vi "Programa Vent.vi"() -> ()   [LabVIEW 2021]
uses:
  4c7040a6-f012-4fa6-bc11-eaa48d4a9fce.vi
  <vilib>/Instr/_visa.llb/VISA Configure Serial Port (Instr).vi
panel:
  out "FLUJO":waveform(dbl)(graph)
  in  "Caract. Escalon":bool
  in  "Caract. Rampa":bool
  in  "Comenzar Caracterizacion":bool
  out "VIF":i16=211
  out "VEF":i16=1
  out "PIP":i16=1
  out "BPM":i16=7
  out "T Ciclo Resp.":dbl=9.2 format="%#_2g"
  in  "Modo Asistido":bool
  out "Fecha y Hora":timestamp=timestamp(3714054510.5922894 s since 1904-01-01) format="%<%X\n%x>T"
  out "PRESIÓN":waveform(dbl)(graph)
  in  "T. Espiración (s)":dbl=3.0 min=1.0 max=5.0 step=0.25
  in  "T. Plateau (s)":dbl=0.5 min=0.0 max=1.0 step=0.1
  in  "Comenzar Respiración":bool
  in  "Volumen deseado":dbl=350.0 min=100.0 max=2000.0 step=10.0
  in  "Presión Soporte\n (Volumen control)":dbl=20.0 min=10.0 max=60.0 step=1.0
  in  "PEEP deseado":dbl=5.0 min=0.0 max=20.0 step=1.0
  in  "Porcentaje Válvula":dbl=50.0 min=0.0 max=100.0 step=1.0
  out "Serial Write":string="0.000000,50.000000,20.000000,5.000000,350.000000,3000.000000,500.000000,0.000000,0.000000,0.000000,0.000000\r\n"
  out "Volumen-Ins":i16=211
  out "Flujo":i16
  out "PEEP":i16=4
  out "Serial Read":string="Presion: 1.42,Peep: 3.57,Presion_soporte: 20,Flujo: -0.35,Volumen deseado: 350, Volumen inspiracion: 211.01,PIP: 1.00,VEF: 1.00,VIF: 211.00,T_muestreo: 4.00, PWM Out: 5000, Timer_Count_0: 0, Etapa_Res: 0, Derivada_Presion: 0.00, duracion_ciclo: 9200.00, BPM: 6.52, PWM_Caract: 0, T. Trans_Caract: 0.00, MV: 0.00, String: 0.000000,50.000000,20.000000,5.000000,350.000000,3000.000000,500.000000,0.000000,0.000000,0.000000,0.000000\r\r\n"
  in  "stop":bool
  # "Ventilador Mecánico de Emergencia"
  # "Modo de Operación"
  # "Volumen\nControl"
  # "GRÁFICOS"
  # "Seccion de Datos:"
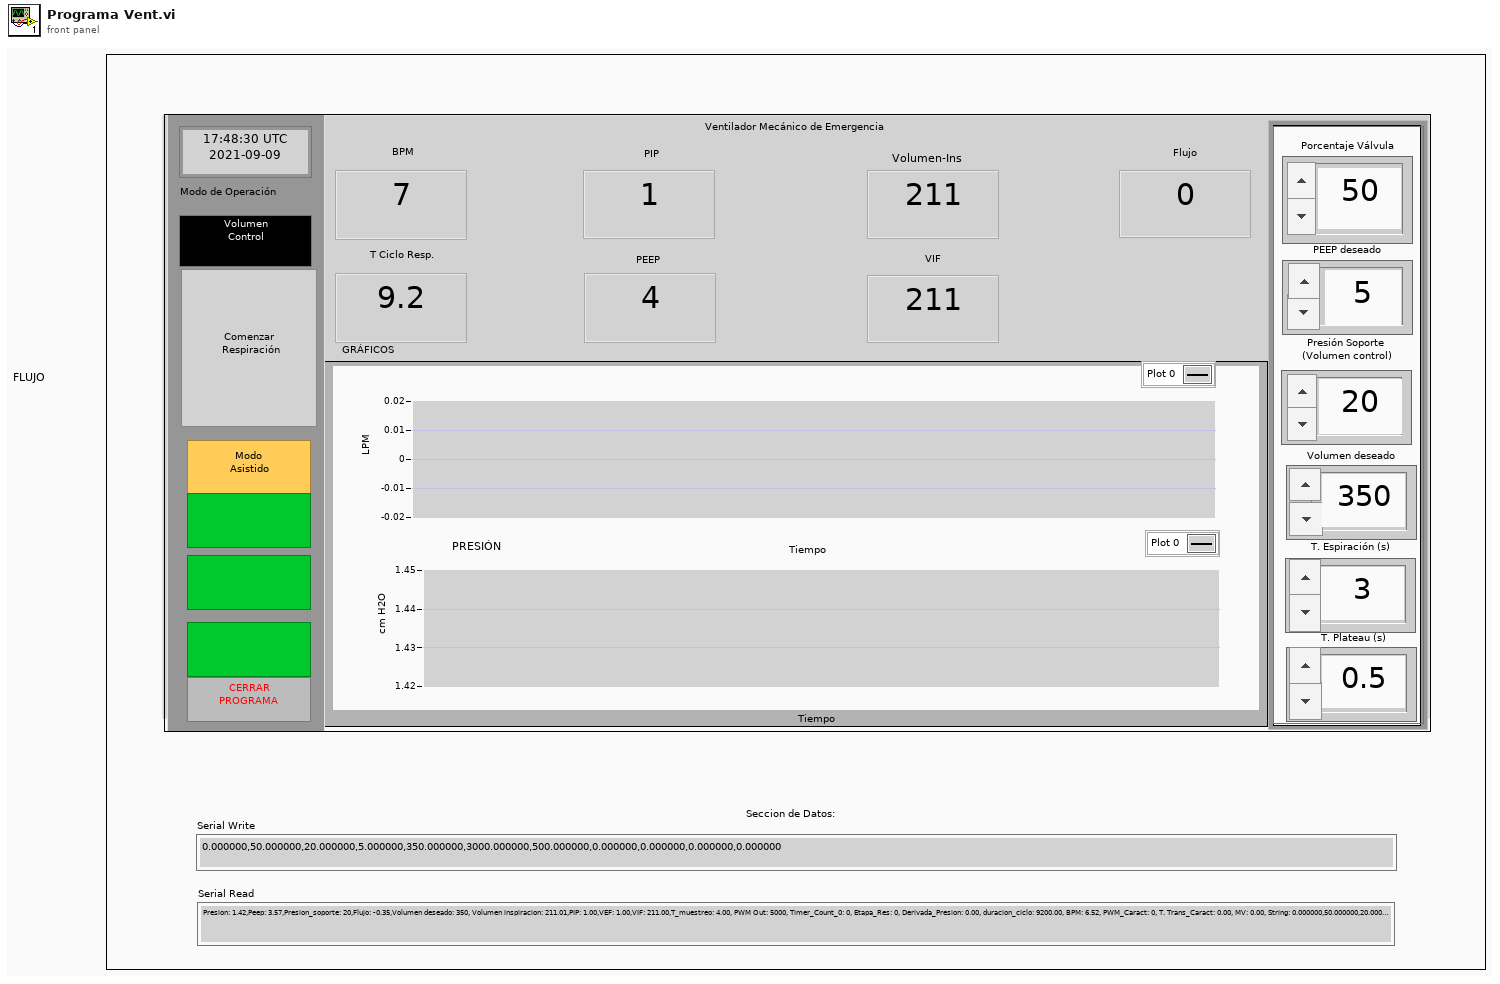
[diagram p1: front panel]
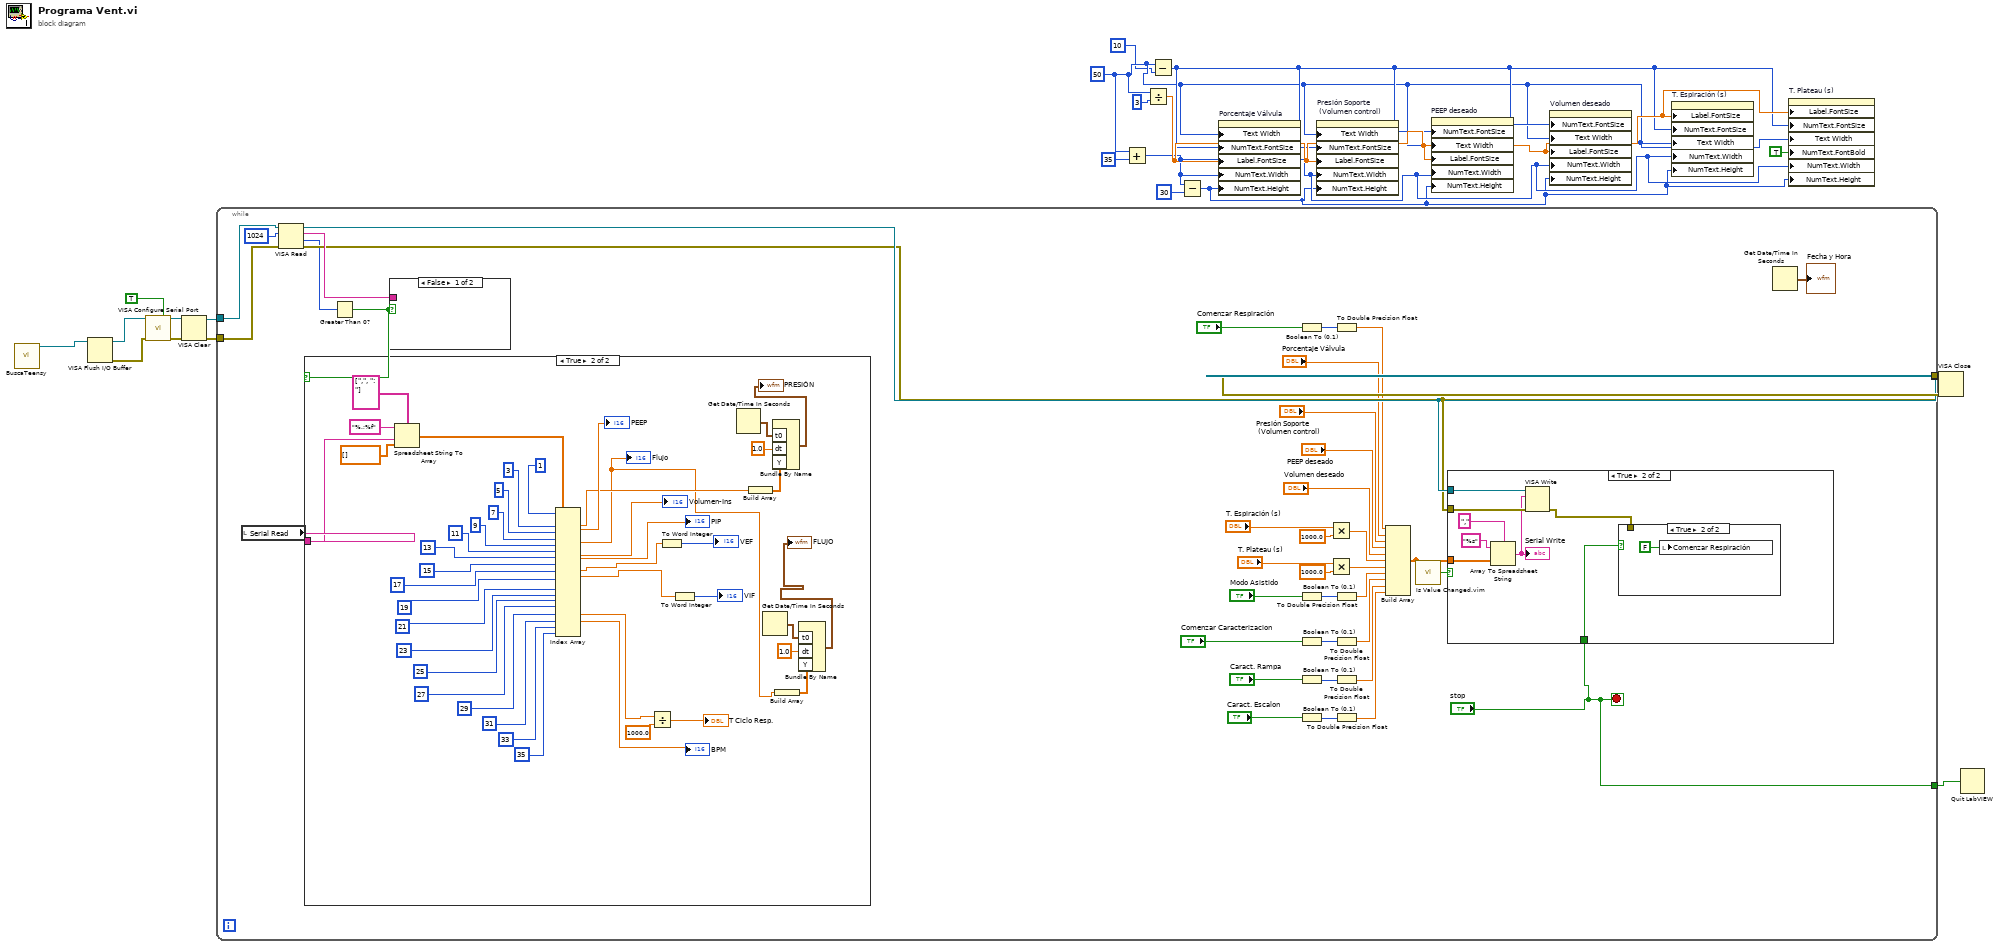
[diagram p0: block diagram]
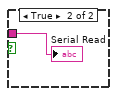
[diagram p3: hidden frame]
diagram:
  w7 = u32 50 ("Numeric Text.Size:Height")
  n1 = call "BuscaTeensy.vi"() -> ("VISA resource name out"=w12:refnum<visa-resource-name>)  [unwired: 15 in]
  n2 = VISA Flush I/O Buffer(VISA resource name=w12) -> (VISA resource name out=w14:refnum<visa-resource-name>, error out=w13:errorcluster)  [unwired: 2 in]
  n3 = call-poly "VISA Configure Serial Port"("VISA resource name"=w14, "Enable Termination\nChar (T)"=TRUE ("Enable Termination\nChar (T)"), "error in (no error)"=w13) -> ("VISA resource name out"=w18:refnum<visa-resource-name>, "error out"=w17:errorcluster)  [unwired: 11 in]
  n4 = VISA Clear(VISA resource name=w18, error in (no error)=w17) -> (VISA resource name out=w16:refnum<visa-resource-name>, error out=w15:errorcluster)
  n5 = while {
    tunnel: [w57] -> w20
    tunnel: [w56] -> w19
    tunnel: w16 -> [w55]
    tunnel: w15 -> [w54]
    tunnel: ["stop"] -> w1
    stop <- "stop" stop-if-true
    n6 = local read "Serial Read"() -> (w58:string)
    n7 = VISA Read(VISA resource name=w55, byte count=u32 1024, error in (no error)=w54) -> (VISA resource name out=w57:refnum<visa-resource-name>, read buffer=w59:string, return count=w52:u32, error out=w56:errorcluster)
    n8 = Greater Than 0?(x=w52) -> (x > 0?=w51:bool)
    n9 = case shown="True" w51 {
      tunnel: w58 -> [_ w100]
      frame False {
      }
      frame True {
        n10 = Spreadsheet String To Array(delimiter (Tab)=string[] [",", ": "], format string="%.;%f", spreadsheet string=w100, array type (2D Dbl)=dbl[] []) -> (array=w99:dbl[])
        n11 = Index Array(array=w99, index #1=1 ("index"), index #2=3 ("index"), index #3=5 ("index"), index #4=7 ("index"), index #5=9 ("index"), index #6=11 ("index"), index #7=13 ("index"), index #8=15 ("index"), index #9=17 ("index"), index #10=19 ("index"), index #11=21 ("index"), index #12=23 ("index"), index #13=25 ("index"), index #14=27 ("index"), index #15=29 ("index"), index #16=31 ("index"), index #17=33 ("index"), index #18=35 ("index")) -> (element #1=w67:dbl, element #2=→"PEEP":dbl, element #4=w60:dbl, element #6=→"Volumen-Ins":dbl, element #7=→"PIP":dbl, element #8=w72:dbl, element #9=w73:dbl, element #15=w76:dbl, element #16=→"BPM":dbl)  [unwired: 9 out]
        "Flujo" <- w60
        n12 = Divide(x=w76, y=1000.0) -> (x/y=→"T Ciclo Resp.":dbl)
        n13 = To Word Integer(number=w72) -> (16bit integer=→"VEF":i16)
        n14 = To Word Integer(number=w73) -> (16bit integer=→"VIF":i16)
        n15 = Get Date/Time In Seconds() -> (seconds since 1Jan1904=w69:timestamp)
        n16 = Build Array(w67) -> (w66:dbl[])
        n17 = Get Date/Time In Seconds() -> (seconds since 1Jan1904=w64:timestamp)
        n18 = Bundle By Name("t0"=w69, "dt"=1.0, "Y"=w66) -> (→"PRESIÓN":waveform(dbl))  [unwired: 1 in]
        n19 = Build Array(w60) -> (w62:dbl[])
        n20 = Bundle By Name("t0"=w64, "dt"=1.0, "Y"=w62) -> (→"FLUJO":waveform(dbl))  [unwired: 1 in]
      }
    }
    n21 = case shown="False" w51 {
      tunnel: w59 -> [_ w104]
      frame False {
      }
      frame True {
        "Serial Read" <- w104
      }
    }
    n22 = Boolean To (0,1)(Boolean="Comenzar Respiración") -> (0, 1=w49:i16)
    n23 = Boolean To (0,1)(Boolean="Modo Asistido") -> (0, 1=w34:i16)
    n24 = Boolean To (0,1)(Boolean="Comenzar Caracterizacion") -> (0, 1=w31:i16)
    n25 = Boolean To (0,1)(Boolean="Caract. Rampa") -> (0, 1=w29:i16)
    n26 = Boolean To (0,1)(Boolean="Caract. Escalon") -> (0, 1=w27:i16)
    n27 = Multiply(x="T. Espiración (s)", y=1000.0) -> (x*y=w40:dbl)
    n28 = Multiply(x="T. Plateau (s)", y=1000.0) -> (x*y=w37:dbl)
    n29 = To Double Precision Float(number=w49) -> (double precision float=w48:dbl)
    n30 = To Double Precision Float(number=w34) -> (double precision float=w33:dbl)
    n31 = To Double Precision Float(number=w31) -> (double precision float=w26:dbl)
    n32 = To Double Precision Float(number=w29) -> (double precision float=w25:dbl)
    n33 = To Double Precision Float(number=w27) -> (double precision float=w24:dbl)
    n34 = Build Array(w48, "Porcentaje Válvula", "Presión Soporte\n (Volumen control)", "PEEP deseado", "Volumen deseado", w40, w37, w33, w26, w25, w24) -> (w47:dbl[])
    n35 = call "Is Value Changed.vim"("value"=w47) -> ("changed or first call?"=w50:bool)
    n36 = case shown="True" w50 {
      tunnel: w57 -> [_ w110]
      tunnel: w56 -> [_ w109]
      tunnel: w47 -> [_ w107]
      tunnel: "stop" -> [_ w105]
      frame False {
      }
      frame True {
        n37 = Array To Spreadsheet String(delimiter (Tab)=",", array=w107, 3:"%s" ("format string")) -> (spreadsheet string=w108:string)
        "Serial Write" <- w108
        n38 = VISA Write(VISA resource name=w110, write buffer=w108, error in (no error)=w109) -> (error out=w106:errorcluster)  [unwired: 2 out]
        n39 = case shown="True" w105 {
          tunnel: w106 -> [_ _]
          frame False {
          }
          frame True {
            n40 = local write "Comenzar Respiración"(FALSE ("Comenzar Respiración")) -> ()
          }
        }
      }
    }
    n41 = Get Date/Time In Seconds() -> (seconds since 1Jan1904=→"Fecha y Hora":timestamp)
  }
  n42 = Add(x=w7, y=u32 35) -> (x+y=w5:u32)
  n43 = Divide(x=w7, y=u32 3) -> (x/y=w9:dbl)
  n44 = Subtract(x=w7, y=u32 10 ("x")) -> (x-y=w8:u32)
  n45 = Subtract(x=w5, y=u32 30) -> (x-y=w3:u32)
  n46 = property on="Porcentaje Válvula" class="DigNum (strict)"("Text Width"=w7, "NumText.FontSize"=w8, "Label.FontSize"=w9, "NumText.Width"=w5, "NumText.Height"=w3) -> ()  [unwired: 2 in, 2 out]
  n47 = property on="Presión Soporte\n (Volumen control)" class="DigNum (strict)"("Text Width"=w7, "NumText.FontSize"=w8, "Label.FontSize"=w9, "NumText.Width"=w5, "NumText.Height"=w3) -> ()  [unwired: 2 in, 2 out]
  n48 = property on="PEEP deseado" class="DigNum (strict)"("NumText.FontSize"=w8, "Text Width"=w7, "Label.FontSize"=w9, "NumText.Width"=w5, "NumText.Height"=w3) -> ()  [unwired: 2 in, 2 out]
  n49 = property on="Volumen deseado" class="DigNum (strict)"("NumText.FontSize"=w8, "Text Width"=w7, "Label.FontSize"=w9, "NumText.Width"=w5, "NumText.Height"=w3) -> ()  [unwired: 2 in, 2 out]
  n50 = property on="T. Espiración (s)" class="DigNum (strict)"("Label.FontSize"=w9, "NumText.FontSize"=w8, "Text Width"=w7, "NumText.Width"=w5, "NumText.Height"=w3) -> ()  [unwired: 2 in, 2 out]
  n51 = property on="T. Plateau (s)" class="DigNum (strict)"("Label.FontSize"=w9, "NumText.FontSize"=w8, "Text Width"=w7, "NumText.FontBold"=TRUE ("Numeric Text.Font:Bold"), "NumText.Width"=w5, "NumText.Height"=w3) -> ()  [unwired: 2 in, 2 out]
  n52 = VISA Close(VISA resource name=w20, error in (no error)=w19) -> ()  [unwired: 1 out]
  n53 = Quit LabVIEW(quit? (T)=w1) -> ()
